vi "String to auto test.vi"() -> ()   [LabVIEW 2017]
panel:
  out "Array":dbl[](array[numeric])
  in  "Load":bool
  in  "Save":bool
  in  "Process":bool
  in  "String":string="d5,f6,r2,"
  out "Direction":string[](array[string])
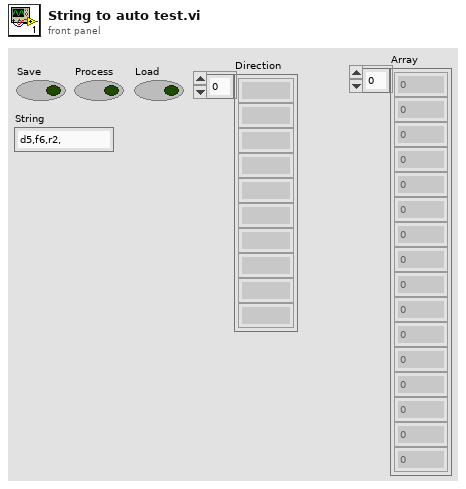
[diagram p1: front panel]
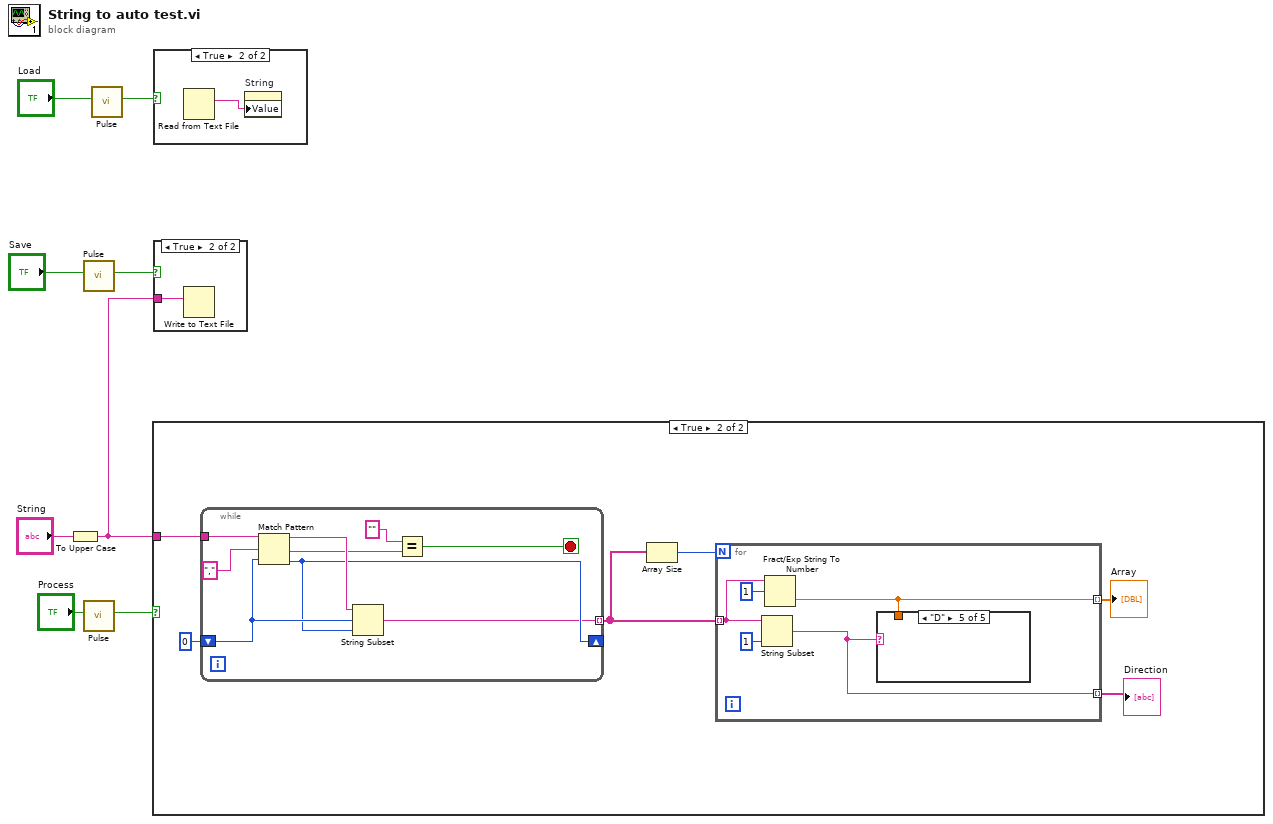
[diagram p0: block diagram]
diagram:
  n1 = To Upper Case(1:"String") -> (0:w1:string)
  n2 = call "Pulse.vi"("Input"="Save") -> ("Output"=w2:bool)  [unwired: 10 in]
  n3 = call "Pulse.vi"("Input"="Process") -> ("Output"=w7:bool)  [unwired: 10 in]
  n4 = call "Pulse.vi"("Input"="Load") -> ("Output"=w3:bool)  [unwired: 10 in]
  n5 = case shown="True" w7 {
    tunnel: w1 -> [_ w13]
    frame False {
    }
    frame True {
      n6 = while {
        tunnel: w13 -> [w28]
        shift-right: [w25] -> _
        shift-left: 0 ("offset past match") -> [w26]
        tunnel: [w24] -> w11 mode=indexing
        stop <- w21 stop-if-true
        n7 = Match Pattern(string=w28, regular expression=",", offset (0)=w26) -> (before substring=w27:string, after substring=w23:string, offset past match=w25:i32)  [unwired: 1 out]
        n8 = String Subset(string=w27, offset (0)=w26, length (rest)=w25) -> (substring=w24:string)
        n9 = Equal?(x="", y=w23) -> (x = y?=w21:bool)
      }
      n10 = Array Size(array=w11) -> (size(s)=w12:i32)
      n11 = for {
        N: w12 -> [_]
        tunnel: w11 -> [w17] mode=indexing
        tunnel: [w15] -> w9 mode=indexing
        tunnel: [w18] -> w10 mode=indexing
        n12 = String Subset(string=w17, length (rest)=1 ("length (rest)")) -> (substring=w18:string)  [unwired: 1 in]
        n13 = Fract/Exp String To Number(string=w17, offset=1) -> (number=w15:dbl)  [unwired: 2 in, 1 out]
        n14 = case shown="\"D\"" w18 {
          tunnel: w15 -> [_ _ _ _ _]
          frame "F", Default {
          }
          frame "B" {
          }
          frame "R" {
          }
          frame "L" {
          }
          frame "D" {
          }
        }
      }
      "Direction" <- w10
      "Array" <- w9
    }
  }
  n15 = case shown="True" w3 {
    frame False {
    }
    frame True {
      n16 = Read from Text File() -> (text=w29:string)  [unwired: 4 in, 3 out]
      n17 = property on="String" class="Str"("Value"=w29) -> ()  [unwired: 2 in, 2 out]
    }
  }
  n18 = case shown="True" w2 {
    tunnel: w1 -> [_ w30]
    frame False {
    }
    frame True {
      n19 = Write to Text File(text=w30) -> ()  [unwired: 3 in, 3 out]
    }
  }
